vi "String to Array Test.vi"(8 "Error In":errorcluster) -> (0 "Error Out":errorcluster)   [LabVIEW 2023, in "Test.lvlib"]
uses:
  Test.lvlib
  <vilib>/addons/_JKI Toolkits/Caraya/classes/Assert/Assert.lvclass
  <vilib>/addons/_JKI Toolkits/Caraya/classes/Assert/Assert Equal Value_Variant.vi
  <vilib>/addons/_JKI Toolkits/Caraya/classes/Test/Test.lvclass
  File Path Operations/File and Path Operations.lvlib
panel:
  # "STRING TO ARRAY TEST"
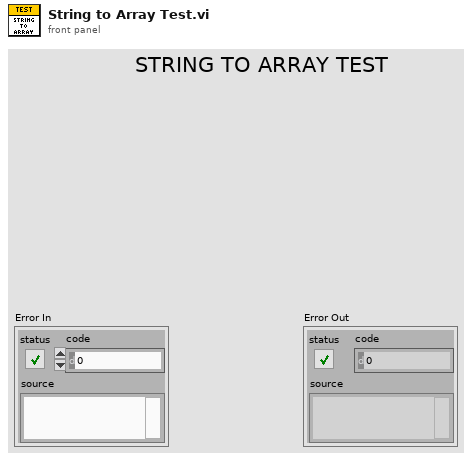
[diagram p1: front panel]
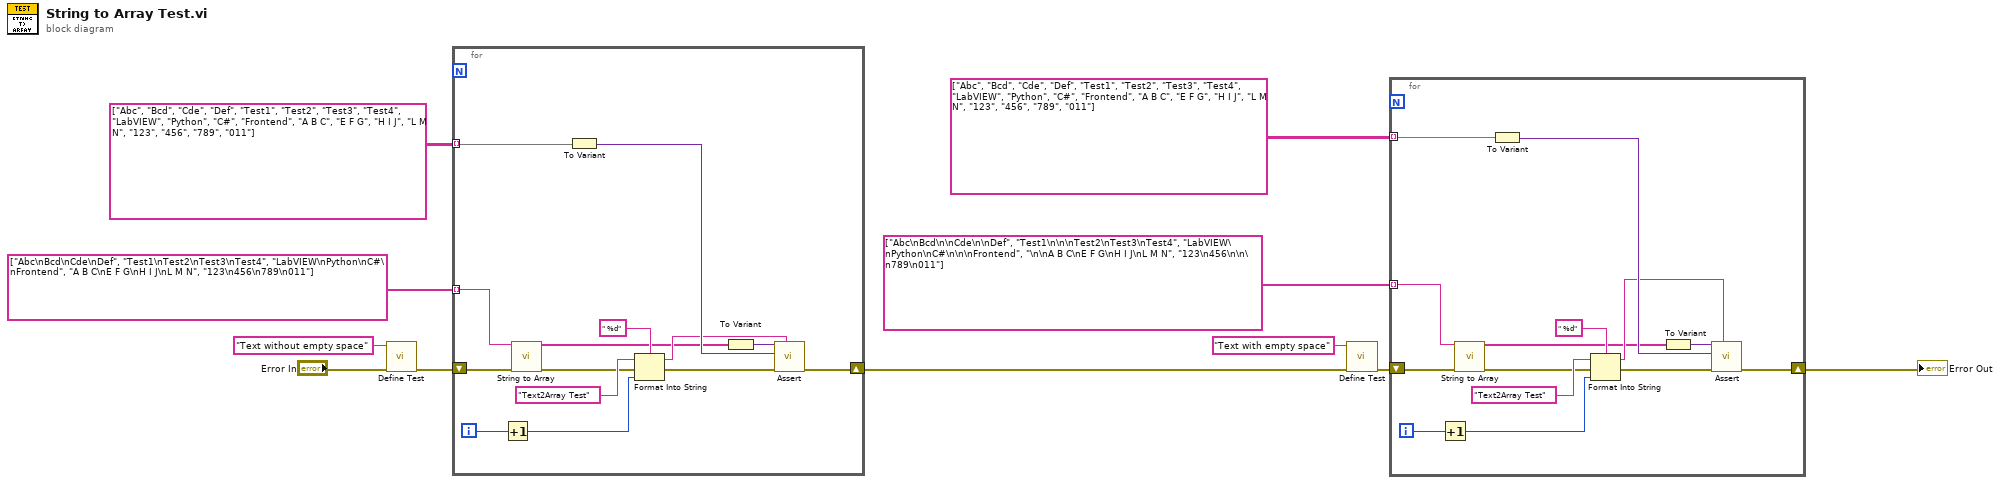
[diagram p0: block diagram]
diagram:
  n1 = call <vilib>:"Define Test.vi"("error in (no error)"="Error In", "Label (VI Title)"="Text without empty space") -> ("error out"=w9:errorcluster)  [unwired: 8 in, 1 out]
  n2 = for {
    shift-right: [w16] -> w4
    shift-left: w9 -> [w15]
    tunnel: string[] ["Abc\nBcd\nCde\nDef", "Test1\nTest2\nTest3\nTest4", "LabVIEW\nPython\nC#\nFrontend", "A B C\nE F G\nH I J\nL M N", "123\n456\n789\n011"] ("Input Array") -> [w12] mode=indexing
    tunnel: string[][] [["Abc", "Bcd", "Cde", "Def"], ["Test1", "Test2", "Test3", "Test4"], ["LabVIEW", "Python", "C#", "Frontend"], ["A B C", "E F G", "H I J", "L M N"], ["123", "456", "789", "011"]] ("Input Array") -> [w17] mode=indexing
    i -> [w21]
    n3 = Increment(x=w21) -> (x+1=w18:i32)
    n4 = call "String to Array.vi"("Input String"=w12, "Error In"=w15) -> ("Array of Strings"=w13:string[], "Error Out"=w14:errorcluster)  [unwired: 12 in]
    n5 = To Variant(anything=w17) -> (Variant=w25:variant)
    n6 = Format Into String(format string=" %d", initial string="Text2Array Test" ("Label"), error in=w14, w18) -> (resulting string=w19:string, error out=w23:errorcluster)
    n7 = To Variant(anything=w13) -> (Variant=w24:variant)
    n8 = call-poly <vilib>:"Assert.vi"("Label"=w19, "error in (no error)"=w23, "Y"=w25, "X"=w24) -> ("error out"=w16:errorcluster)  [unwired: 6 in, 1 out]
  }
  n9 = call <vilib>:"Define Test.vi"("error in (no error)"=w4, "Label (VI Title)"="Text with empty space") -> ("error out"=w5:errorcluster)  [unwired: 8 in, 1 out]
  n10 = for {
    shift-right: [w31] -> w3
    shift-left: w5 -> [w30]
    tunnel: string[] ["Abc\nBcd\n\nCde\n\nDef", "Test1\n\n\nTest2\nTest3\nTest4", "LabVIEW\nPython\nC#\n\n\nFrontend", "\n\nA B C\nE F G\nH I J\nL M N", "123\n456\n\n\n789\n011"] ("Input Array") -> [w27] mode=indexing
    tunnel: string[][] [["Abc", "Bcd", "Cde", "Def"], ["Test1", "Test2", "Test3", "Test4"], ["LabVIEW", "Python", "C#", "Frontend"], ["A B C", "E F G", "H I J", "L M N"], ["123", "456", "789", "011"]] ("Input Array") -> [w26] mode=indexing
    i -> [w35]
    n11 = Increment(x=w35) -> (x+1=w32:i32)
    n12 = call "String to Array.vi"("Input String"=w27, "Error In"=w30) -> ("Array of Strings"=w28:string[], "Error Out"=w29:errorcluster)  [unwired: 12 in]
    n13 = To Variant(anything=w26) -> (Variant=w39:variant)
    n14 = Format Into String(format string=" %d", initial string="Text2Array Test" ("Label"), error in=w29, w32) -> (resulting string=w33:string, error out=w37:errorcluster)
    n15 = To Variant(anything=w28) -> (Variant=w38:variant)
    n16 = call-poly <vilib>:"Assert.vi"("Label"=w33, "error in (no error)"=w37, "Y"=w39, "X"=w38) -> ("error out"=w31:errorcluster)  [unwired: 6 in, 1 out]
  }
  "Error Out" <- w3
